vi "Test Assert Array Not Empty.vi"(8 "error in (no error)":errorcluster) -> (0 "error out":errorcluster)   [LabVIEW 2013]
uses:
  classes/Test/Test.lvclass
  classes/Assert/Assert.lvclass
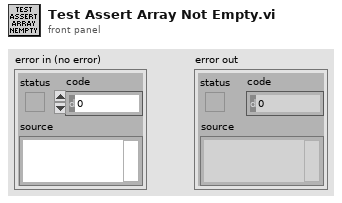
[diagram p1: front panel]
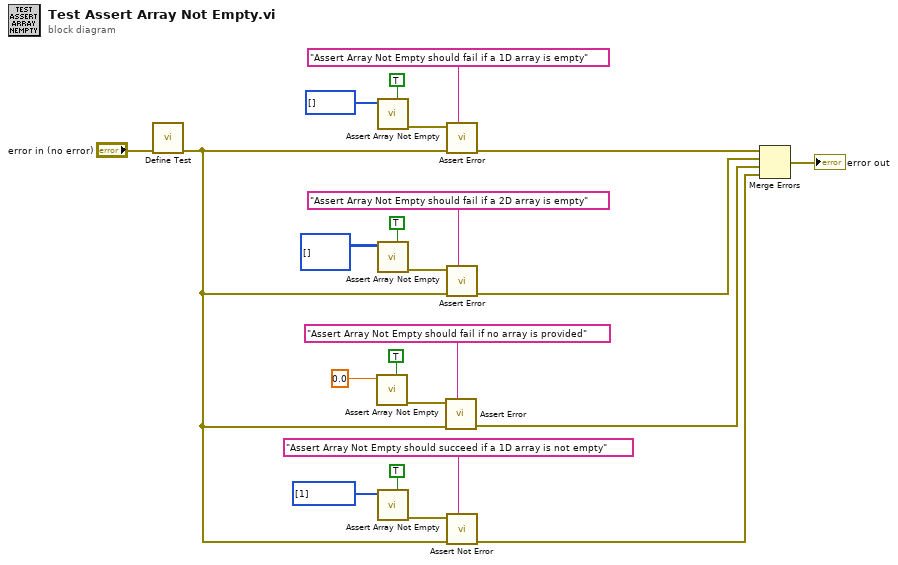
[diagram p0: block diagram]
diagram:
  n1 = call "Define Test.vi"("error in (no error)"="error in (no error)") -> ("error out"=w5:errorcluster)  [unwired: 9 in, 1 out]
  n2 = call "Assert Array Not Empty.vi"("Assert Only? (F)"=TRUE, "Array"=0.0 ("element")) -> ("error out"=w11:errorcluster)  [unwired: 8 in, 1 out]
  n3 = call "Assert Array Not Empty.vi"("Assert Only? (F)"=TRUE, "Array"=i32[] []) -> ("error out"=w23:errorcluster)  [unwired: 8 in, 1 out]
  n4 = call "Assert Array Not Empty.vi"("Assert Only? (F)"=TRUE, "Array"=i32[][] []) -> ("error out"=w15:errorcluster)  [unwired: 8 in, 1 out]
  n5 = call "Assert Array Not Empty.vi"("Assert Only? (F)"=TRUE, "Array"=i32[] [1]) -> ("error out"=w6:errorcluster)  [unwired: 8 in, 1 out]
  n6 = call "Assert Error.vi"("Label"="Assert Array Not Empty should fail if no array is provided", "error in (no error)"=w5, "Error?"=w11) -> ("error out"=w9:errorcluster)  [unwired: 7 in, 1 out]
  n7 = call "Assert Error.vi"("Label"="Assert Array Not Empty should fail if a 1D array is empty", "error in (no error)"=w5, "Error?"=w23) -> ("error out"=w19:errorcluster)  [unwired: 7 in, 1 out]
  n8 = call "Assert Error.vi"("Label"="Assert Array Not Empty should fail if a 2D array is empty", "error in (no error)"=w5, "Error?"=w15) -> ("error out"=w14:errorcluster)  [unwired: 7 in, 1 out]
  n9 = call "Assert Not Error.vi"("Label"="Assert Array Not Empty should succeed if a 1D array is not empty", "error in (no error)"=w5, "Not Error?"=w6) -> ("error out"=w4:errorcluster)  [unwired: 7 in, 1 out]
  n10 = Merge Errors(w19, w14, w9, w4) -> (→"error out":errorcluster)
